vi "control functions to channels.vi"(11 "control functions":T1[](array[typedef]) {"output range"."output low" format="%.2f"; "output range"."output high" format="%.2f"}) -> (3 "channels":refnum<class "TBM channel.lvclass">[](array[class]))   [LabVIEW 2013, in "configuration tests.lvlib" / "TEST CONFIGURATION.lvclass"]
uses:
  TEST CONFIGURATION.lvclass
  <vilib>/NI/Tag Bus Module Framework/channel/TBM channel.lvclass
  control module configuration.ctl
  gains.ctl
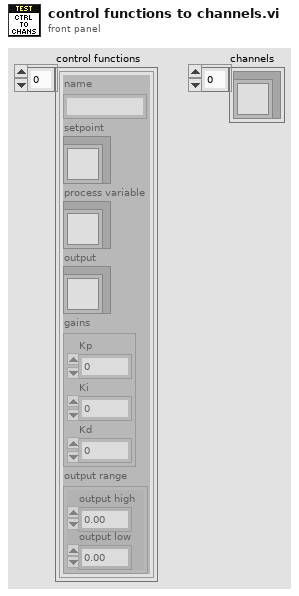
[diagram p1: front panel]
types:
  T1 = typedef "configuration tests.lvlib/TEST CONFIGURATION.lvclass/control module configuration.ctl" = cluster{"name":string, "setpoint":refnum<class "TBM channel.lvclass">, "process variable":refnum<class "TBM channel.lvclass">, "output":refnum<class "TBM channel.lvclass">, "gains":T2, "output range":cluster{"output high":dbl, "output low":dbl}}
  T2 = typedef "configuration tests.lvlib/TEST CONFIGURATION.lvclass/gains.ctl" = cluster{"Kp":dbl, "Ki":dbl, "Kd":dbl}
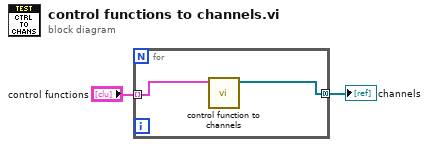
[diagram p0: block diagram]
diagram:
  n1 = for {
    tunnel: "control functions" -> [w4] mode=indexing
    tunnel: [w3] -> w2 mode=concatenating
    n2 = call "control function to channels.vi"("control module configuration"=w4) -> ("channels"=w3:refnum<class "TBM channel.lvclass">[])  [unwired: 10 in]
  }
  "channels" <- w2
